vi "rs3 Advanced get depth control3.vi"(8 "error in (no error)":errorcluster, 10 "mode":i32, 11 "device in":u64) -> (0 "error out 2":errorcluster, 1 "error":u64, 2 "depth control":T1, 3 "Dev out":u64)   [LabVIEW 2017, in "libRealSense3.lvlib"]
doc: "Opens communication to a specific RealSense Device."
uses:
  libRealSense3.lvlib
  realsense2.dll
panel:
  # "RS3 Adv. Get Depth Control 2"
  # "(C) 2017 Intel Corp.,  AGJ"
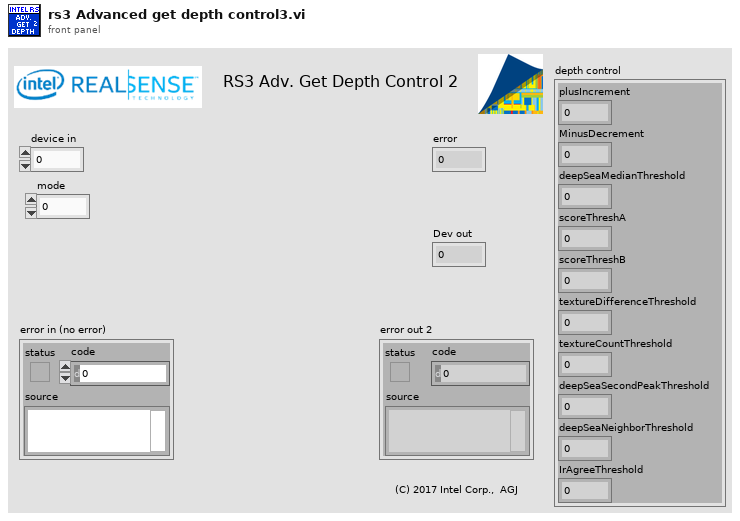
[diagram p1: front panel]
types:
  T1 = cluster{"plusIncrement":u32, "MinusDecrement":u32, "deepSeaMedianThreshold":u32, "scoreThreshA":u32, "scoreThreshB":u32, "textureDifferenceThreshold":u32, "textureCountThreshold":u32, "deepSeaSecondPeakThreshold":u32, "deepSeaNeighborThreshold":u32, "IrAgreeThreshold":u32}
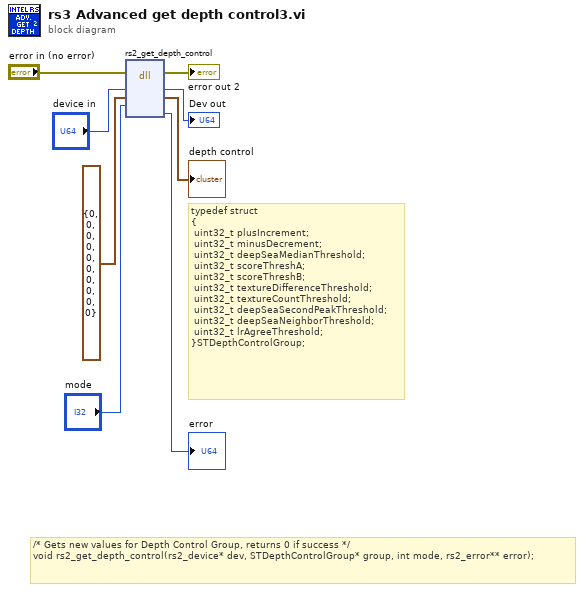
[diagram p0: block diagram]
diagram:
  # "/* Gets new values for Depth Control Group, returns 0 if success */\nvoid rs2_get_depth_control(rs2_device* dev, STDepthControlGroup* group, int mode, rs2_error** error);"
  # "typedef struct\n{\n\tuint32_t plusIncrement;\n\tuint32_t minusDecrement;\n\tuint32_t deepSeaMedianThreshold;\n\tuint32_t scoreThreshA;\n\tuint32_t scoreThreshB;\n\tuint32_t textureDifferenceThreshold;\n\tuint32_t textureCountThreshold;\n\tuint32_t deepSeaSecondPeakThreshold;\n\tuint32_t deepSeaNeighborThreshold;\n\tuint32_t lrAgreeThreshold;\n}STDepthControlGroup;"
  n1 = dll-call lib="C:/Users/agrunnet/Documents/libRealSense6/realsense2.dll" fn="rs2_get_depth_control"(error in="error in (no error)", "device"="device in", "depth control"=T1 {"plusIncrement"=0, "MinusDecrement"=0, "deepSeaMedianThreshold"=0, "scoreThreshA"=0, "scoreThreshB"=0, "textureDifferenceThreshold"=0, "textureCountThreshold"=0, "deepSeaSecondPeakThreshold"=0, "deepSeaNeighborThreshold"=0, "IrAgreeThreshold"=0}, "mode"="mode") -> (error out=→"error out 2":errorcluster, "device"=→"Dev out":u64, "depth control"=→"depth control":T1, "error"=→"error":u64)  [unwired: 5 in, 1 out]
